vi "Frame.Settings.vi"(6 "Action":enum8{"Get", "Set"}(ring), 8 "error in (no error)":errorcluster, 10 "Frame.Settings":T1={"ID"=0, "Disable Transmission"=FALSE, "Disable Transmission Ref"=18446744073709551615, "Transmit Trigger"=enum."Channel value change", "Transmit Trigger Ref"=18446744073709551615} {"Transmit Trigger Ref" format="%.0x"; "Disable Transmission Ref" format="%.0x"}, 11 "Item Ref in":T2 format="%.0x") -> (0 "error out":errorcluster, 2 "Frame.Settings":T1={"ID"=0, "Disable Transmission"=FALSE, "Disable Transmission Ref"=18446744073709551615, "Transmit Trigger"=enum."Channel value change", "Transmit Trigger Ref"=18446744073709551615} {"Transmit Trigger Ref" format="%.0x"; "Disable Transmission Ref" format="%.0x"}, 3 "Item Ref out":T2 format="%.0x")   [LabVIEW 2023, in "J1939 Addon Shared.lvlib"]
uses:
  J1939 Addon Shared.lvlib
  <vilib>/NI VeriStand/Custom Device API/Custom Device Item Ref.ctl
  Types/Frame.Settings.ctl
  Types/Outgoing Event Trigger Types.ctl
  Constants.vi
  <vilib>/NI VeriStand/Custom Device API/Set Item Property (Dependent Node Pointer).vi
  <vilib>/NI VeriStand/Custom Device API/Set Item Property (U32).vi
  <vilib>/NI VeriStand/Custom Device API/Set Item Property (Boolean).vi
  <vilib>/NI VeriStand/Custom Device API/Get Item Property (Dependent Node Pointer).vi
  <vilib>/NI VeriStand/Custom Device API/Get Item Property (U32).vi
  <vilib>/NI VeriStand/Custom Device API/Get Item Property (Boolean).vi
  <vilib>/NI VeriStand/Custom Device API/Custom Device API.lvlib
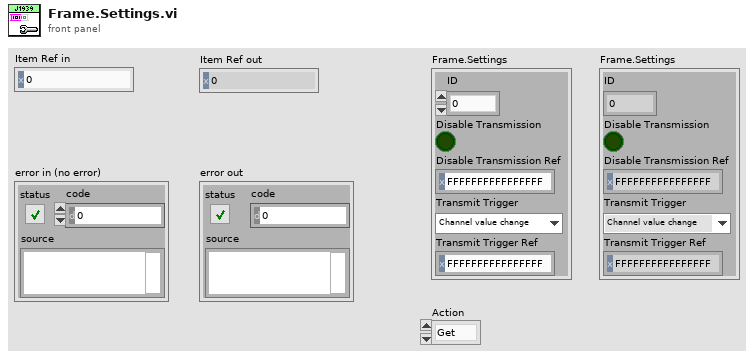
[diagram p1: front panel]
types:
  T1 = typedef "J1939 Addon Shared.lvlib/Frame.Settings.ctl" = cluster{"ID":u32, "Disable Transmission":bool, "Disable Transmission Ref":T2, "Transmit Trigger":T3, "Transmit Trigger Ref":T2}
  T2 = typedef "Custom Device API.lvlib/Custom Device Item Ref.ctl" = u64
  T3 = typedef "J1939 Addon Shared.lvlib/Outgoing Event Trigger Types.ctl" = enum16{"Channel value change", "Trigger channel (not zero)", "Channel value change or trigger channel (not zero)", "Trigger channel (any value change)", "Channel value change or trigger channel (any value change)"}
  T4 = typedef "Custom Device API.lvlib/Custom Device Item Info.ctl" = cluster{"Name":string, "Is Channel":bool, "GUID":string, "Is Waveform":bool}
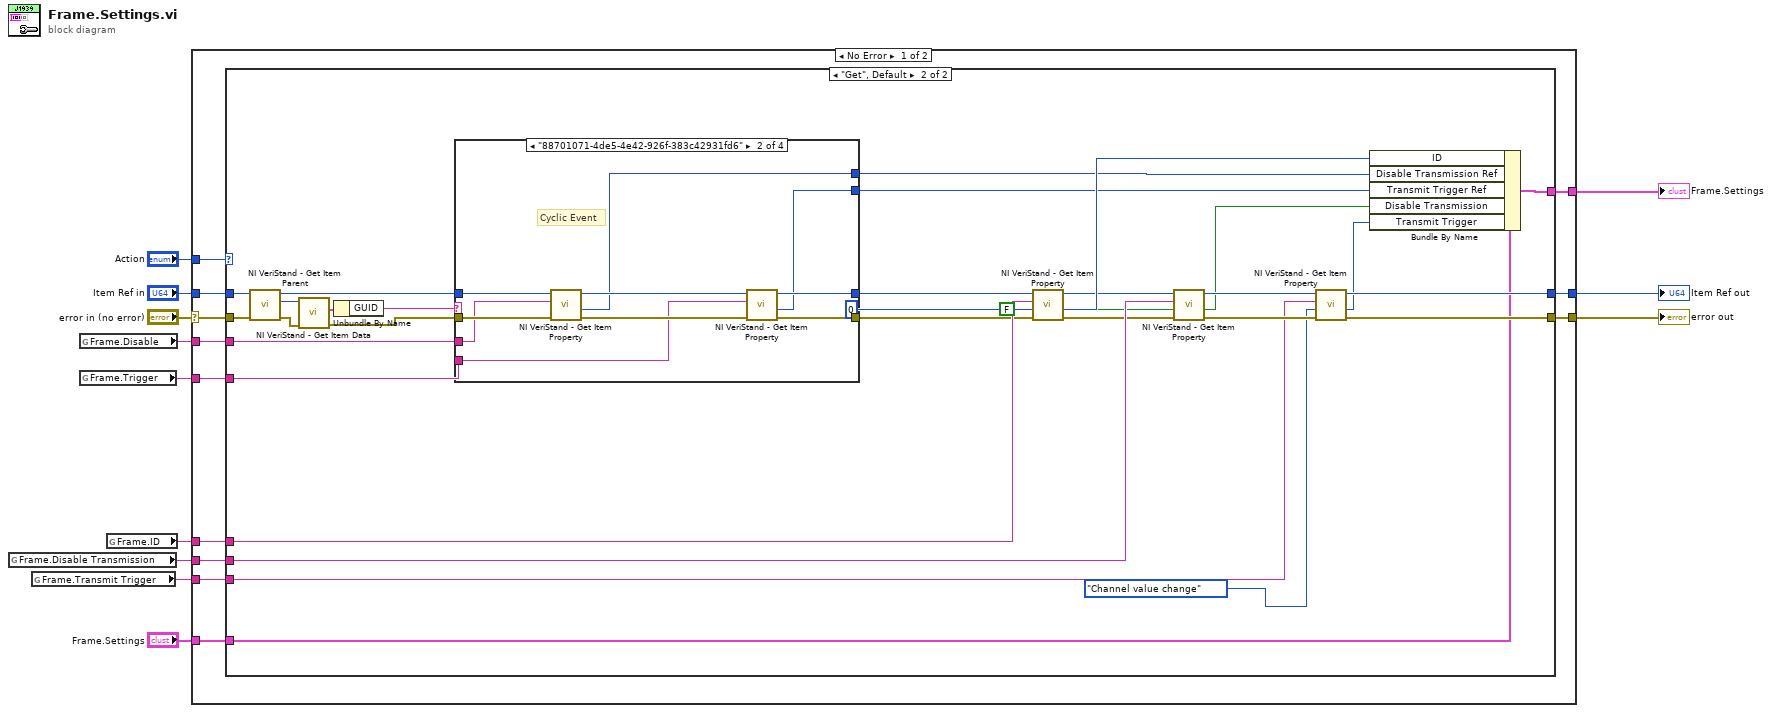
[diagram p0: block diagram]
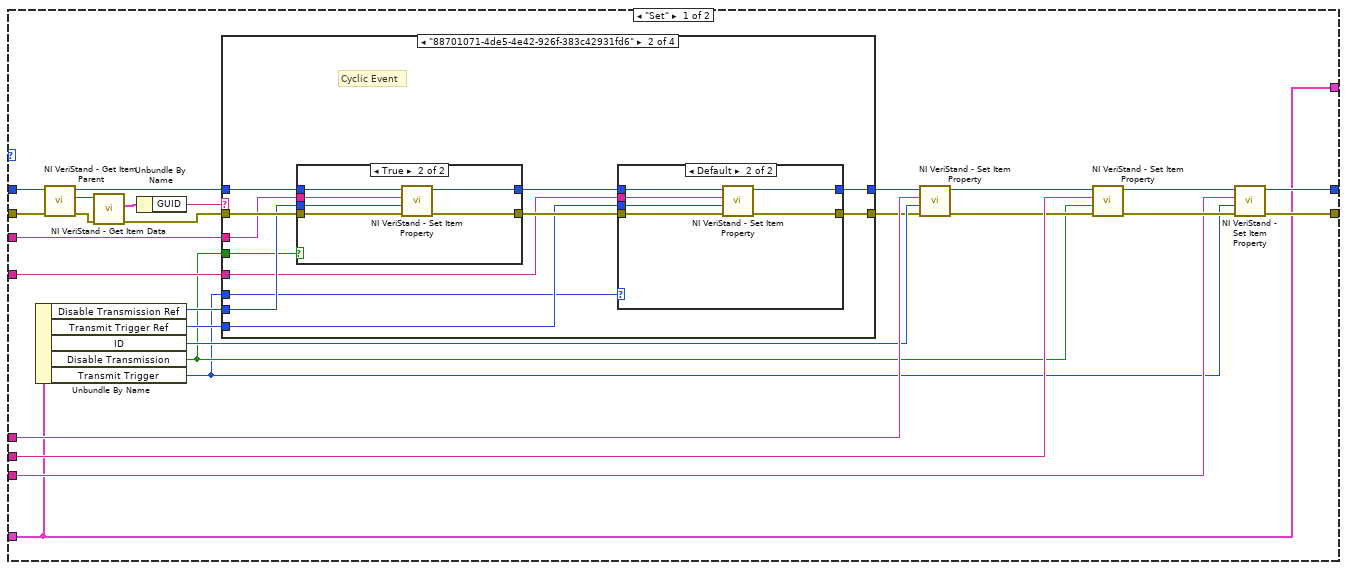
[diagram p2: hidden frame]
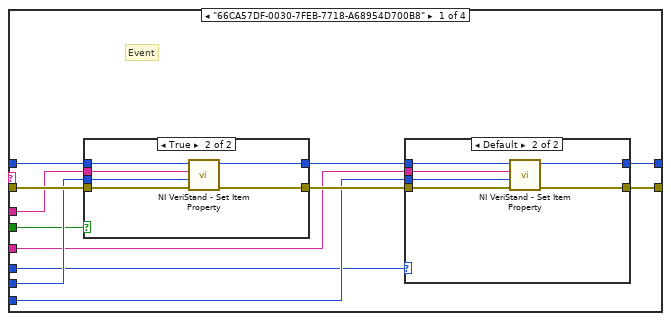
[diagram p3: hidden frame]
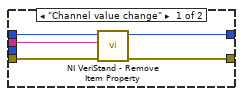
[diagram p4: hidden frame]
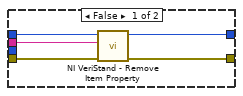
[diagram p5: hidden frame]
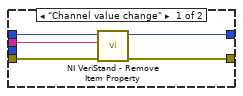
[diagram p6: hidden frame]
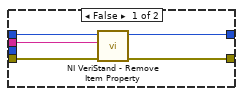
[diagram p7: hidden frame]
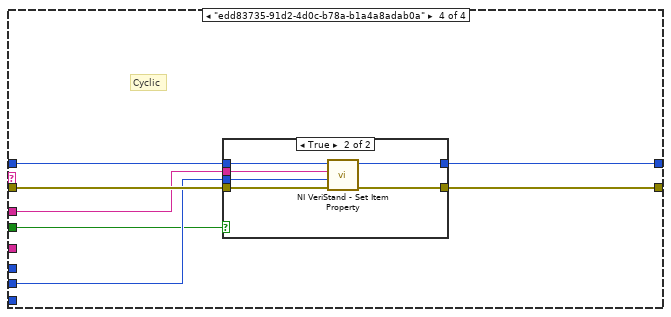
[diagram p9: hidden frame]
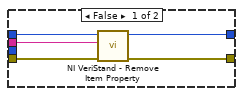
[diagram p10: hidden frame]
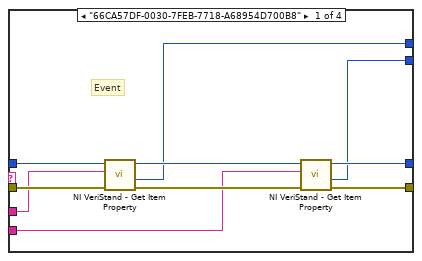
[diagram p11: hidden frame]
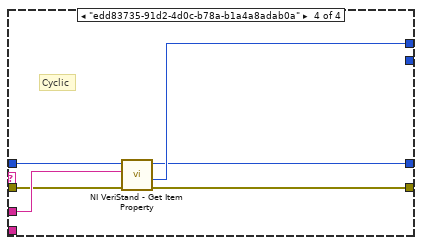
[diagram p13: hidden frame]
diagram:
  n1 = global read "Constants.vi" "Frame.Disable Transmission"() -> (w4:string)
  n2 = global read "Constants.vi" "Frame.Transmit Trigger"() -> (w5:string)
  n3 = global read "Constants.vi" "Frame.Disable"() -> (w10:string)
  n4 = global read "Constants.vi" "Frame.Trigger"() -> (w9:string)
  n5 = global read "Constants.vi" "Frame.ID"() -> (w11:string)
  n6 = case shown="No Error" "error in (no error)" {
    selector: "error in (no error)" -> [w15 w199]
    tunnel: "Item Ref in" -> [w24 w198]
    tunnel: w11 -> [w23 _]
    tunnel: w10 -> [w22 _]
    tunnel: w9 -> [w21 _]
    tunnel: [w20 w199] -> w8
    tunnel: [w19 w198] -> w7
    tunnel: [w18 _] -> w6
    tunnel: w5 -> [w17 _]
    tunnel: w4 -> [w16 _]
    tunnel: "Frame.Settings" -> [w14 _]
    tunnel: "Action" -> [w13 _]
    frame No Error {
      n7 = case shown="\"Get\", Default" w13 {
        tunnel: w24 -> [w37 w149]
        tunnel: w23 -> [w50 w169]
        tunnel: w22 -> [w34 w144]
        tunnel: w21 -> [w33 w143]
        tunnel: [w47 w165] -> w20
        tunnel: [w46 w164] -> w19
        tunnel: [w43 w157] -> w18
        tunnel: w17 -> [w45 w163]
        tunnel: w16 -> [w44 w162]
        tunnel: w15 -> [w36 w146]
        tunnel: w14 -> [w43 w158]
        frame "Set" {
          n8 = Unbundle By Name(w43) -> ("Disable Transmission Ref"=w28:T2, "Transmit Trigger Ref"=w27:T2, "ID"=w42:u32, "Disable Transmission"=w26:bool, "Transmit Trigger"=w25:T3)
          n9 = call <vilib>:"NI VeriStand - Get Item Parent.vi"("error in (no error)"=w36, "Item Ref in"=w37) -> ("error out"=w32:errorcluster, "Parent Ref"=w39:T2, "Item Ref out"=w38:T2)  [unwired: 6 in, 1 out]
          n10 = call <vilib>:"NI VeriStand - Get Item Data.vi"("error in (no error)"=w32, "Item Ref in"=w39) -> ("error out"=w35:errorcluster, "Item Info"=w40:T4)  [unwired: 8 out]
          n11 = Unbundle By Name(w40) -> ("GUID"=w41:string)
          n12 = case shown="\"88701071-4de5-4e42-926f-383c42931fd6\"" w41 {
            tunnel: w35 -> [w62 w96 w120 w127]
            tunnel: [w52 w86 w120 w122] -> w31
            tunnel: w34 -> [w61 w95 _ w125]
            tunnel: w33 -> [w55 w89 _ _]
            tunnel: w38 -> [w60 w94 w119 w124]
            tunnel: [w53 w87 w119 w123] -> _
            tunnel: w28 -> [w59 w93 _ w126]
            tunnel: w27 -> [w56 w90 _ _]
            tunnel: w26 -> [w58 w92 _ w121]
            tunnel: w25 -> [w51 w85 _ _]
            frame "66CA57DF-0030-7FEB-7718-A68954D700B8" {
              # "Event"
              n13 = case shown="True" w58 {
                tunnel: [w74 w84] -> w54
                tunnel: [w75 w83] -> w57
                tunnel: w62 -> [w76 w82]
                tunnel: w61 -> [w77 w81]
                tunnel: w60 -> [w78 w80]
                tunnel: w59 -> [_ w79]
                frame False {
                  n14 = call <vilib>:"NI VeriStand - Remove Item Property.vi"("error in (no error)"=w76, "Property Name"=w77, "Item Ref in"=w78) -> ("error out"=w75:errorcluster, "Item Ref out"=w74:T2)  [unwired: 6 in, 1 out]
                }
                frame True {
                  n15 = call-poly <vilib>:"NI VeriStand - Set Item Property.vi"("error in (no error)"=w82, "Dependent Node Ref"=w79, "Property Name"=w81, "Item Ref in"=w80) -> ("error out"=w83:errorcluster, "Item Ref out"=w84:T2)  [unwired: 5 in, 1 out]
                }
              }
              n16 = case shown="Default" w51 {
                tunnel: [w63 w73] -> w53
                tunnel: [w64 w72] -> w52
                tunnel: w57 -> [w65 w71]
                tunnel: w55 -> [w66 w70]
                tunnel: w54 -> [w67 w69]
                tunnel: w56 -> [_ w68]
                frame "Channel value change" {
                  n17 = call <vilib>:"NI VeriStand - Remove Item Property.vi"("error in (no error)"=w65, "Property Name"=w66, "Item Ref in"=w67) -> ("error out"=w64:errorcluster, "Item Ref out"=w63:T2)  [unwired: 6 in, 1 out]
                }
                frame Default {
                  n18 = call-poly <vilib>:"NI VeriStand - Set Item Property.vi"("error in (no error)"=w71, "Dependent Node Ref"=w68, "Property Name"=w70, "Item Ref in"=w69) -> ("error out"=w72:errorcluster, "Item Ref out"=w73:T2)  [unwired: 5 in, 1 out]
                }
              }
            }
            frame "88701071-4de5-4e42-926f-383c42931fd6" {
              # "Cyclic Event"
              n19 = case shown="True" w92 {
                tunnel: [w108 w118] -> w88
                tunnel: [w109 w117] -> w91
                tunnel: w96 -> [w110 w116]
                tunnel: w95 -> [w111 w115]
                tunnel: w94 -> [w112 w114]
                tunnel: w93 -> [_ w113]
                frame False {
                  n20 = call <vilib>:"NI VeriStand - Remove Item Property.vi"("error in (no error)"=w110, "Property Name"=w111, "Item Ref in"=w112) -> ("error out"=w109:errorcluster, "Item Ref out"=w108:T2)  [unwired: 6 in, 1 out]
                }
                frame True {
                  n21 = call-poly <vilib>:"NI VeriStand - Set Item Property.vi"("error in (no error)"=w116, "Dependent Node Ref"=w113, "Property Name"=w115, "Item Ref in"=w114) -> ("error out"=w117:errorcluster, "Item Ref out"=w118:T2)  [unwired: 5 in, 1 out]
                }
              }
              n22 = case shown="Default" w85 {
                tunnel: [w97 w107] -> w87
                tunnel: [w98 w106] -> w86
                tunnel: w91 -> [w99 w105]
                tunnel: w89 -> [w100 w104]
                tunnel: w88 -> [w101 w103]
                tunnel: w90 -> [_ w102]
                frame "Channel value change" {
                  n23 = call <vilib>:"NI VeriStand - Remove Item Property.vi"("error in (no error)"=w99, "Property Name"=w100, "Item Ref in"=w101) -> ("error out"=w98:errorcluster, "Item Ref out"=w97:T2)  [unwired: 6 in, 1 out]
                }
                frame Default {
                  n24 = call-poly <vilib>:"NI VeriStand - Set Item Property.vi"("error in (no error)"=w105, "Dependent Node Ref"=w102, "Property Name"=w104, "Item Ref in"=w103) -> ("error out"=w106:errorcluster, "Item Ref out"=w107:T2)  [unwired: 5 in, 1 out]
                }
              }
            }
            frame "F09FE425-7E71-8634-77FE-097EFBD4E192", Default {
              # "SinglePoint"
            }
            frame "edd83735-91d2-4d0c-b78a-b1a4a8adab0a" {
              # "Cyclic"
              n25 = case shown="True" w121 {
                tunnel: [w128 w138] -> w123
                tunnel: [w129 w137] -> w122
                tunnel: w127 -> [w130 w136]
                tunnel: w125 -> [w131 w135]
                tunnel: w124 -> [w132 w134]
                tunnel: w126 -> [_ w133]
                frame False {
                  n26 = call <vilib>:"NI VeriStand - Remove Item Property.vi"("error in (no error)"=w130, "Property Name"=w131, "Item Ref in"=w132) -> ("error out"=w129:errorcluster, "Item Ref out"=w128:T2)  [unwired: 6 in, 1 out]
                }
                frame True {
                  n27 = call-poly <vilib>:"NI VeriStand - Set Item Property.vi"("error in (no error)"=w136, "Dependent Node Ref"=w133, "Property Name"=w135, "Item Ref in"=w134) -> ("error out"=w137:errorcluster, "Item Ref out"=w138:T2)  [unwired: 5 in, 1 out]
                }
              }
            }
          }
          n28 = call-poly <vilib>:"NI VeriStand - Set Item Property.vi"("error in (no error)"=w31, "Value"=w42, "Property Name"=w50, "Item Ref in"=w37) -> ("error out"=w30:errorcluster, "Item Ref out"=w29:T2)  [unwired: 5 in, 1 out]
          n29 = call-poly <vilib>:"NI VeriStand - Set Item Property.vi"("error in (no error)"=w30, "Value"=w26, "Property Name"=w44, "Item Ref in"=w29) -> ("error out"=w48:errorcluster, "Item Ref out"=w49:T2)  [unwired: 5 in, 1 out]
          n30 = call-poly <vilib>:"NI VeriStand - Set Item Property.vi"("error in (no error)"=w48, "Value"=w25, "Property Name"=w45, "Item Ref in"=w49) -> ("error out"=w47:errorcluster, "Item Ref out"=w46:T2)  [unwired: 5 in, 1 out]
        }
        frame "Get", Default {
          n31 = call <vilib>:"NI VeriStand - Get Item Parent.vi"("error in (no error)"=w146, "Item Ref in"=w149) -> ("error out"=w150:errorcluster, "Parent Ref"=w151:T2, "Item Ref out"=w142:T2)  [unwired: 6 in, 1 out]
          n32 = call <vilib>:"NI VeriStand - Get Item Data.vi"("error in (no error)"=w150, "Item Ref in"=w151) -> ("error out"=w152:errorcluster, "Item Info"=w153:T4)  [unwired: 8 out]
          n33 = Unbundle By Name(w153) -> ("GUID"=w154:string)
          n34 = case shown="\"88701071-4de5-4e42-926f-383c42931fd6\"" w154 {
            tunnel: w152 -> [w177 w187 w191 w195]
            tunnel: [w176 w186 w191 w194] -> w145
            tunnel: w144 -> [w175 w185 _ w197]
            tunnel: w143 -> [w174 w184 _ _]
            tunnel: w142 -> [w173 w183 w190 w196]
            tunnel: [w172 w182 w190 w192] -> w141
            tunnel: [w171 w181 _ w193] -> w140
            tunnel: [w170 w180 _ _] -> w139
            frame "66CA57DF-0030-7FEB-7718-A68954D700B8" {
              # "Event"
              n35 = call-poly <vilib>:"NI VeriStand - Get Item Property.vi"("error in (no error)"=w177, "Property Name"=w175, "Item Ref in"=w173) -> ("error out"=w178:errorcluster, "Dependent Node Ref"=w171:T2, "Item Ref out"=w179:T2)  [unwired: 5 in, 1 out]
              n36 = call-poly <vilib>:"NI VeriStand - Get Item Property.vi"("error in (no error)"=w178, "Property Name"=w174, "Item Ref in"=w179) -> ("error out"=w176:errorcluster, "Dependent Node Ref"=w170:T2, "Item Ref out"=w172:T2)  [unwired: 5 in, 1 out]
            }
            frame "88701071-4de5-4e42-926f-383c42931fd6" {
              # "Cyclic Event"
              n37 = call-poly <vilib>:"NI VeriStand - Get Item Property.vi"("error in (no error)"=w187, "Property Name"=w185, "Item Ref in"=w183) -> ("error out"=w188:errorcluster, "Dependent Node Ref"=w181:T2, "Item Ref out"=w189:T2)  [unwired: 5 in, 1 out]
              n38 = call-poly <vilib>:"NI VeriStand - Get Item Property.vi"("error in (no error)"=w188, "Property Name"=w184, "Item Ref in"=w189) -> ("error out"=w186:errorcluster, "Dependent Node Ref"=w180:T2, "Item Ref out"=w182:T2)  [unwired: 5 in, 1 out]
            }
            frame "F09FE425-7E71-8634-77FE-097EFBD4E192", Default {
              # "SinglePoint"
            }
            frame "edd83735-91d2-4d0c-b78a-b1a4a8adab0a" {
              # "Cyclic"
              n39 = call-poly <vilib>:"NI VeriStand - Get Item Property.vi"("error in (no error)"=w195, "Property Name"=w197, "Item Ref in"=w196) -> ("error out"=w194:errorcluster, "Dependent Node Ref"=w193:T2, "Item Ref out"=w192:T2)  [unwired: 5 in, 1 out]
            }
          }
          n40 = call-poly <vilib>:"NI VeriStand - Get Item Property.vi"("error in (no error)"=w145, "Default Value"=u32 0, "Property Name"=w169, "Item Ref in"=w141) -> ("error out"=w148:errorcluster, "Value"=w161:u32, "Item Ref out"=w147:T2)  [unwired: 4 in, 1 out]
          n41 = call-poly <vilib>:"NI VeriStand - Get Item Property.vi"("error in (no error)"=w148, "Default Value"=FALSE, "Property Name"=w162, "Item Ref in"=w147) -> ("error out"=w166:errorcluster, "Value"=w159:bool, "Item Ref out"=w167:T2)  [unwired: 4 in, 1 out]
          n42 = call-poly <vilib>:"NI VeriStand - Get Item Property.vi"("error in (no error)"=w166, "Default Value"=Outgoing_Event_Trigger_Types."Channel value change" ("Transmit Trigger"), "Property Name"=w163, "Item Ref in"=w167) -> ("error out"=w165:errorcluster, "Value"=w160:u32, "Item Ref out"=w164:T2)  [unwired: 4 in, 1 out]
          n43 = Bundle By Name(cluster=w158, "ID"=w161, "Disable Transmission Ref"=w140, "Transmit Trigger Ref"=w139, "Disable Transmission"=w159, "Transmit Trigger"=w160) -> (w157:T1)
        }
      }
    }
    frame Error {
    }
  }
  "Item Ref out" <- w7
  "error out" <- w8
  "Frame.Settings" <- w6
